vi "calculate benchmark.vi"(9 "end":dbl, 10 "middle":dbl, 11 "beginning":dbl) -> (0 "lvjson faster?":bool, 1 "ratio":dbl, 2 "lvjson time":dbl, 3 "i3 time":dbl)   [LabVIEW 2017, in "LVJSON Tests.lvlib"]
uses:
  LVJSON Tests.lvlib
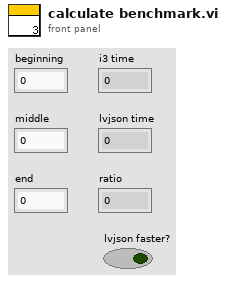
[diagram p1: front panel]
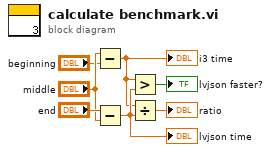
[diagram p0: block diagram]
diagram:
  n1 = Subtract(x="middle", y="beginning") -> (x-y=w5:dbl)
  "i3 time" <- w5
  n2 = Subtract(x="end", y="middle") -> (x-y=w6:dbl)
  "lvjson time" <- w6
  n3 = Greater?(x=w5, y=w6) -> (0:→"lvjson faster?":bool)
  n4 = Divide(x=w5, y=w6) -> (x/y=→"ratio":dbl)
